vi "Color Electrode Box.vi"(8 "error in (no error)":errorcluster, 9 "Electrode Type":string, 10 "Electrode Name":string, 11 "Reference":refnum<vi>) -> (0 "error out":errorcluster)   [LabVIEW 2020, in "Retrieve and Visualize.lvclass"]
uses:
  Retrieve and Visualize.lvclass
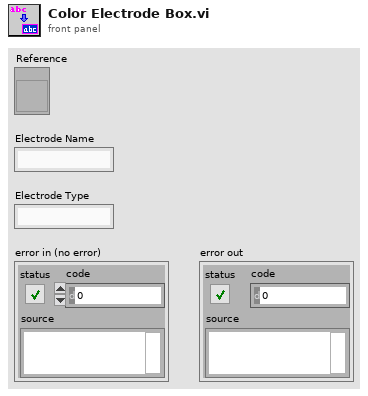
[diagram p1: front panel]
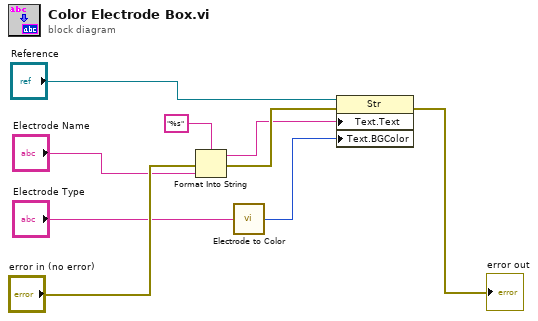
[diagram p0: block diagram]
diagram:
  n1 = Format Into String(format string="%s", error in="error in (no error)", "Electrode Name") -> (resulting string=w6:string, error out=w7:errorcluster)  [unwired: 1 in]
  n2 = call "Electrode to Color.vi"("Electrode Type"="Electrode Type") -> ("Color"=w2:u32)
  n3 = property on="Property Node" class="Str"(reference="Reference", error in=w7, "Text.Text"=w6, "Text.BGColor"=w2) -> (error out=→"error out":errorcluster)  [unwired: 1 out]
